vi "OA Get String.vi"(7 "uiStringLen":u32, 9 "pcStringValue":string, 10 "pcModeParam":string, 11 "pcModeName":string) -> (1 "pcStringValue out":string, 3 "function return":u32)   [LabVIEW 2018, in "AndorSDK.lvlib"]
doc: "EXPNETTYPE unsigned int WINAPI OA_GetString(const char * const pcModeName, const char * const pcModeParam, char * pcStringValue, const unsigned int uiStringLen);"
uses:
  AndorSDK.lvlib
  ATMCD32D.dll
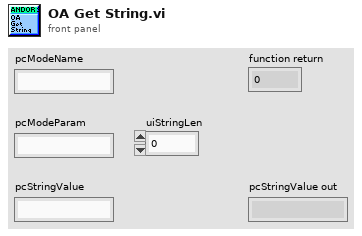
[diagram p1: front panel]
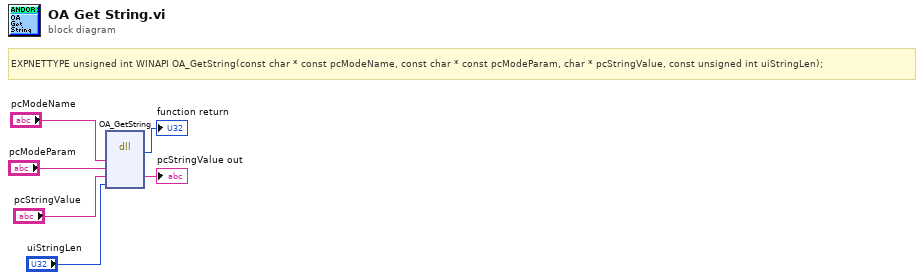
[diagram p0: block diagram]
diagram:
  # "EXPNETTYPE unsigned int WINAPI OA_GetString(const char * const pcModeName, const char * const pcModeParam, char * pcStringValue, const unsigned int uiStringLen);"
  n1 = dll-call lib="PTH2babs E\nPersönliches02 - Arbeit03-HiwijobsLabviewCodelibANDOR\tAndor SDK\nATMCD32D.*" fn="OA_GetString"("pcModeName"="pcModeName", "pcModeParam"="pcModeParam", "pcStringValue"="pcStringValue", "uiStringLen"="uiStringLen") -> (→"function return":u32, "pcStringValue"=→"pcStringValue out":string)  [unwired: 6 in, 2 out]
